vi "OP150ZP_SEALING.vi"(8 "ERRIN":errorcluster caption="entrée d'erreur (pas d'erreur)") -> (0 "ERROUT":errorcluster caption="sortie d'erreur", 2 "SEALING_VALUE":dbl, 3 "IsOK?":bool)   [LabVIEW 2020]
uses:
  <instrlib>/HIOKI BT356X Series/HIOKI BT356X Series.lvlib
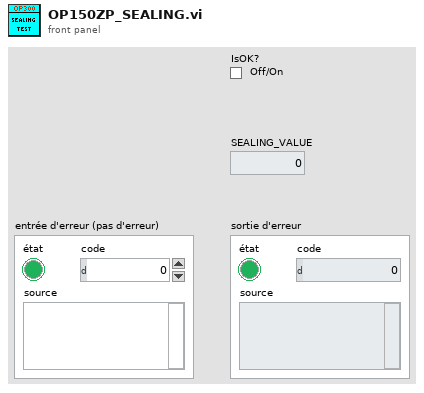
[diagram p1: front panel]
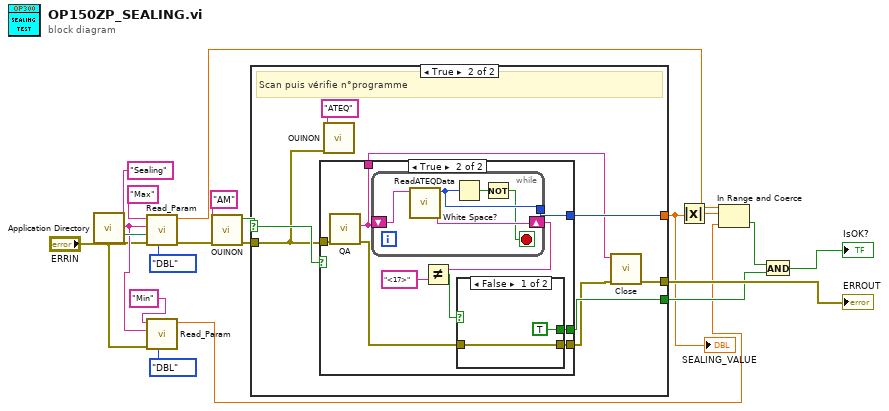
[diagram p0: block diagram]
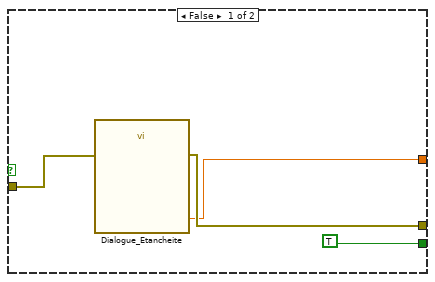
[diagram p2: hidden frame]
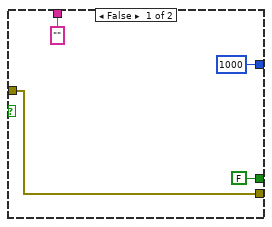
[diagram p3: hidden frame]
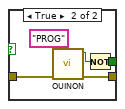
[diagram p4: hidden frame]
diagram:
  w3 = "Sealing" ("section")
  n1 = call <vilib>:"Application Directory.vi"() -> ("Application Directory"=w18:path)
  n2 = call "Read_Param.vi"("Énum"=enum16{"STR", "DBL", "U32"}."DBL", "errin"="ERRIN", "pathin"=w18, "section"=w3, "key"="Max") -> ("error out"=w11:errorcluster, "dbl"=w15:dbl)  [unwired: 2 in, 3 out]
  n3 = call "Read_Param.vi"("Énum"=enum16{"STR", "DBL", "U32"}."DBL", "errin"="ERRIN", "section"=w3, "key"="Min") -> ("dbl"=w1:dbl)  [unwired: 3 in, 4 out]
  n4 = call "OUINON.vi"("errin"=w11, "image"="AM" ("IN")) -> ("error out"=w9:errorcluster, "OUI/NON"=w10:bool)  [unwired: 8 in]
  n5 = case shown="True" w10 {
    selector: w10 -> [_ w28]
    tunnel: [w22 w31] -> w7
    tunnel: [w23 w25] -> w19
    tunnel: [TRUE w30] -> w13
    tunnel: w9 -> [w20 w27]
    frame False {
      n6 = call "Dialogue_Etancheite.vi"("error in (no error)"=w20) -> ("Valeur d'étanchéité"=w22:dbl, "error out"=w23:errorcluster)  [unwired: 16 in, 1 out]
    }
    frame True {
      # "Scan puis vérifie n°programme"
      n7 = case shown="True" w28 {
        tunnel: [1000 ("Valeur") w44] -> w31
        tunnel: [w35 w42] -> w26
        tunnel: [FALSE w41] -> w30
        tunnel: w27 -> [w35 w37]
        tunnel: ["" ("DATAOUT") w36] -> w24
        frame False {
        }
        frame True {
          n8 = call "QA.vi"("ERRIN"=w37) -> ("ERROUT"=w43:errorcluster, "DATAOUT"=w36:string)  [unwired: 9 in]
          n9 = while {
            tunnel: [w49] -> w44
            shift-right: [w47] -> w40
            shift-left: w36 -> [w48]
            stop <- w45 stop-if-true
            n10 = call "ReadATEQData.vi"("Chaîne"=w48) -> ("Prg number"=w47:string, "Valeur"=w49:i32)  [unwired: 7 in, 2 out]
            n11 = White Space?(1:w49) -> (0:w46:bool)
            n12 = Not(x=w46) -> (.not. x?=w45:bool)
          }
          n13 = Not Equal?(x=w40, y="<17>") -> (x != y?=w38:bool)
          n14 = case shown="False" w38 {
            tunnel: w43 -> [w50 w55]
            tunnel: [w50 w54] -> w42
            tunnel: [TRUE w52] -> w41
            frame False {
            }
            frame True {
              n15 = call "OUINON.vi"("errin"=w55, "image"="PROG" ("IN")) -> ("error out"=w54:errorcluster, "OUI/NON"=w53:bool)  [unwired: 8 in]
              n16 = Not(x=w53) -> (.not. x?=w52:bool)
            }
          }
        }
      }
      n17 = call "OUINON.vi"("errin"=w27, "image"="ATEQ" ("IN")) -> ()  [unwired: 8 in, 2 out]
      n18 = call <instrlib>:"Close.vi"("error in (no error)"=w26, "VISA resource name"=w24) -> ("error out"=w25:errorcluster)  [unwired: 9 in]
    }
  }
  "SEALING_VALUE" <- w7
  "ERROUT" <- w19
  n19 = Absolute Value(x=w7) -> (abs(x)=w6:dbl)
  n20 = In Range and Coerce ("Dans la gamme")(upper limit=w15, x=w6, lower limit=w1) -> (In Range?=w14:bool)  [unwired: 1 out]
  n21 = And(x=w14, y=w13) -> (x .and. y?=→"IsOK?":bool)
